vi "GetImage.vi"(0 "XRef":T4, 1 "State In":T3) -> (14 "Image":T2, 15 "Fatal Error Out":T1)   [LabVIEW 2015, in "Index JSON Array.xnode"]
uses:
  Index JSON Array.xnode
  <vilib>/XNodeSupport/XNodeXNodeRef.ctl
  State.ctl
  <vilib>/XNodeSupport/XNodeImage.ctl
  <vilib>/XNodeSupport/XNodeErrorCluster.ctl
  Build Array XNode/dimensions.vi
  Build Array XNode/Build JSON Array.xnode
  <vilib>/XNodeSupport/NI_XNodeSupport.lvlib
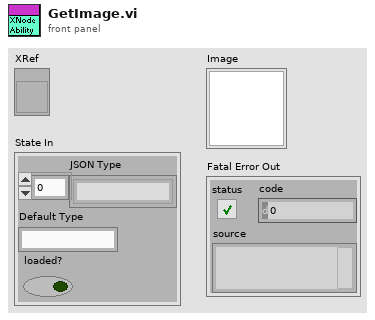
[diagram p1: front panel]
types:
  T1 = typedef "NI_XNodeSupport.lvlib/XNodeErrorCluster.ctl" = errorcluster
  T2 = typedef "NI_XNodeSupport.lvlib/XNodeImage.ctl" = picture
  T3 = typedef "Index JSON Array.xnode/State.ctl" = cluster{"JSON Type":string[], "Default Type":string, "loaded?":bool}
  T4 = typedef "NI_XNodeSupport.lvlib/XNodeXNodeRef.ctl" = refnum<vi>
  T5 = typedef "imagedata.ctl" = cluster{"image type":i32, "image depth":i32, "image":u8[], "mask":u8[], "colors":u32[], "Rectangle":cluster{"left":i16, "top":i16, "right":i16, "bottom":i16}}
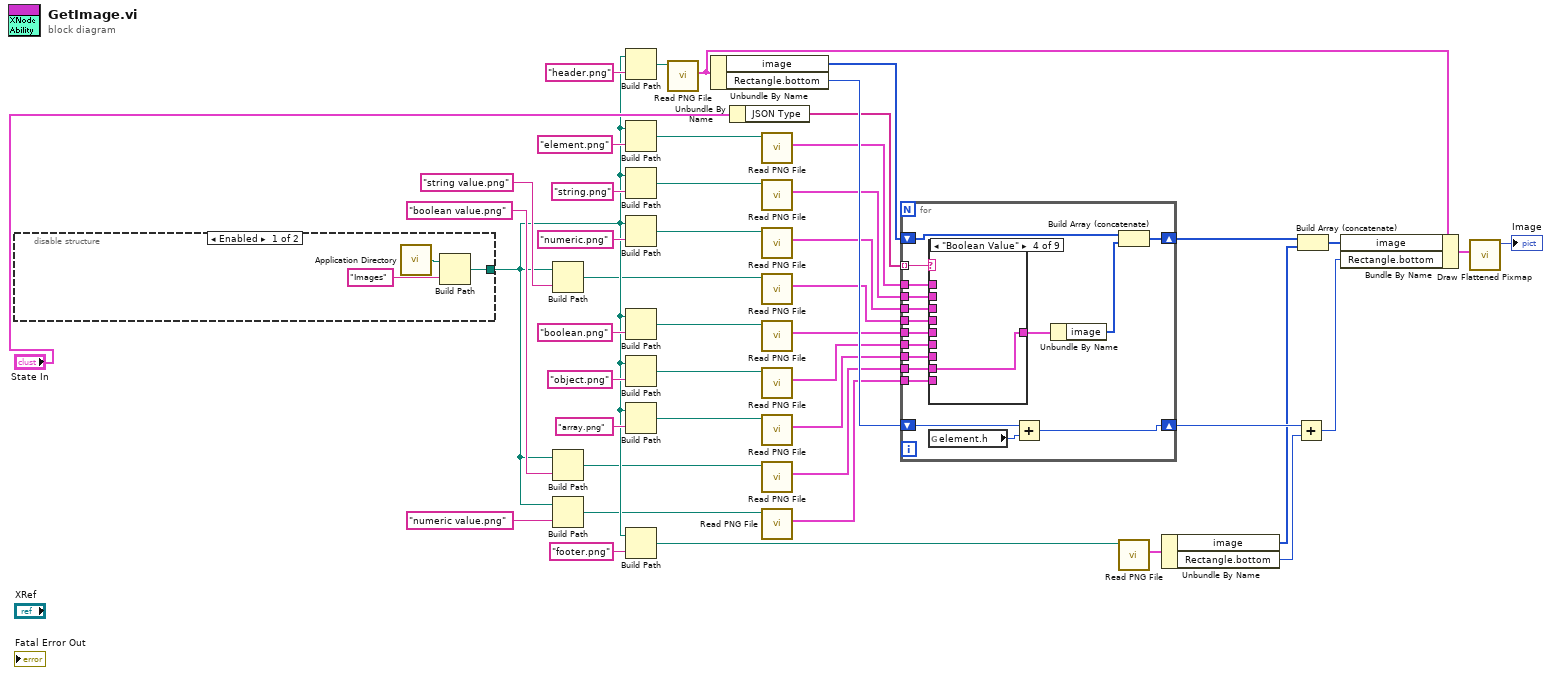
[diagram p0: block diagram]
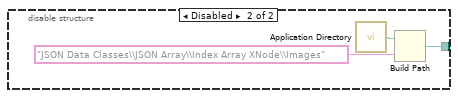
[diagram p10: hidden frame]
diagram:
  n1 = disable-structure shown="Enabled" {
    disable-tunnel: [w48 w51] -> w7
    frame Enabled {
      n2 = call <vilib>:"Application Directory.vi"() -> ("Application Directory"=w47:path)
      n3 = Build Path(base path=w47, name or relative path="Images") -> (appended path=w48:path)
    }
    frame Disabled {
      n4 = call <vilib>:"Application Directory.vi"() -> ("Application Directory"=w50:path)
      n5 = Build Path(base path=w50, name or relative path="JSON Data Classes\\JSON Array\\Index Array XNode\\Images") -> (appended path=w51:path)
    }
  }
  n6 = Build Path(base path=w7, name or relative path="string value.png") -> (appended path=w6:path)
  n7 = Build Path(base path=w7, name or relative path="boolean value.png") -> (appended path=w4:path)
  n8 = Build Path(base path=w7, name or relative path="numeric value.png") -> (appended path=w5:path)
  n9 = Build Path(base path=w7, name or relative path="header.png") -> (appended path=w42:path)
  n10 = Build Path(base path=w7, name or relative path="element.png") -> (appended path=w41:path)
  n11 = Build Path(base path=w7, name or relative path="string.png") -> (appended path=w25:path)
  n12 = Build Path(base path=w7, name or relative path="numeric.png") -> (appended path=w18:path)
  n13 = Build Path(base path=w7, name or relative path="boolean.png") -> (appended path=w16:path)
  n14 = Build Path(base path=w7, name or relative path="object.png") -> (appended path=w14:path)
  n15 = Build Path(base path=w7, name or relative path="array.png") -> (appended path=w15:path)
  n16 = Build Path(base path=w7, name or relative path="footer.png") -> (appended path=w40:path)
  n17 = call <vilib>:"Read PNG File.vi"("path to PNG file"=w42) -> ("image data"=w46:T5)  [unwired: 8 in, 2 out]
  n18 = Unbundle By Name(w46) -> ("image"=w38:u8[], "Rectangle.bottom"=w36:i16)
  n19 = Unbundle By Name("State In") -> ("JSON Type"=w27:string[])
  n20 = call <vilib>:"Read PNG File.vi"("path to PNG file"=w41) -> ("image data"=w23:T5)  [unwired: 8 in, 2 out]
  n21 = call <vilib>:"Read PNG File.vi"("path to PNG file"=w25) -> ("image data"=w24:T5)  [unwired: 8 in, 2 out]
  n22 = call <vilib>:"Read PNG File.vi"("path to PNG file"=w18) -> ("image data"=w17:T5)  [unwired: 8 in, 2 out]
  n23 = call <vilib>:"Read PNG File.vi"("path to PNG file"=w6) -> ("image data"=w3:T5)  [unwired: 8 in, 2 out]
  n24 = call <vilib>:"Read PNG File.vi"("path to PNG file"=w16) -> ("image data"=w13:T5)  [unwired: 8 in, 2 out]
  n25 = call <vilib>:"Read PNG File.vi"("path to PNG file"=w14) -> ("image data"=w11:T5)  [unwired: 8 in, 2 out]
  n26 = call <vilib>:"Read PNG File.vi"("path to PNG file"=w15) -> ("image data"=w12:T5)  [unwired: 8 in, 2 out]
  n27 = call <vilib>:"Read PNG File.vi"("path to PNG file"=w4) -> ("image data"=w1:T5)  [unwired: 8 in, 2 out]
  n28 = call <vilib>:"Read PNG File.vi"("path to PNG file"=w5) -> ("image data"=w2:T5)  [unwired: 8 in, 2 out]
  n29 = for {
    shift-right: [w65] -> w35
    shift-left: w38 -> [w69]
    shift-right: [w66] -> w33
    shift-left: w36 -> [w68]
    tunnel: w27 -> [w64] mode=indexing
    tunnel: w24 -> [w63]
    tunnel: w23 -> [w60]
    tunnel: w17 -> [w59]
    tunnel: w13 -> [w58]
    tunnel: w12 -> [w57]
    tunnel: w11 -> [w56]
    tunnel: w3 -> [w55]
    tunnel: w2 -> [w54]
    tunnel: w1 -> [w53]
    n30 = case shown="\"Boolean Value\"" w64 {
      tunnel: w63 -> [_ _ _ _ w74 _ _ _ _]
      tunnel: [w70 w71 w72 w73 w74 w75 w76 w77 w78] -> w62
      tunnel: w60 -> [w70 _ _ _ _ _ _ _ _]
      tunnel: w59 -> [_ _ _ _ _ w75 _ _ _]
      tunnel: w58 -> [_ _ _ _ _ _ w76 _ _]
      tunnel: w57 -> [_ _ _ _ _ _ _ w77 _]
      tunnel: w56 -> [_ _ _ _ _ _ _ _ w78]
      tunnel: w55 -> [_ w71 _ _ _ _ _ _ _]
      tunnel: w54 -> [_ _ w72 _ _ _ _ _ _]
      tunnel: w53 -> [_ _ _ w73 _ _ _ _ _]
      frame "JSON", Default {
      }
      frame "String Value" {
      }
      frame "Numeric Value" {
      }
      frame "Boolean Value" {
      }
      frame "JSON String" {
      }
      frame "JSON Numeric" {
      }
      frame "JSON Boolean" {
      }
      frame "JSON Array" {
      }
      frame "JSON Object" {
      }
    }
    n31 = global read "dimensions.vi" "element.h"() -> (w67:i16)
    n32 = Add(x=w68, y=w67) -> (x+y=w66:i16)
    n33 = Unbundle By Name(w62) -> ("image"=w61:u8[])
    n34 = Build Array (concatenate)(w69, w61) -> (w65:u8[])
  }
  n35 = call <vilib>:"Read PNG File.vi"("path to PNG file"=w40) -> ("image data"=w45:T5)  [unwired: 8 in, 2 out]
  n36 = Unbundle By Name(w45) -> ("image"=w32:u8[], "Rectangle.bottom"=w31:i16)
  n37 = Add(x=w33, y=w31) -> (x+y=w30:i16)
  n38 = Build Array (concatenate)(w35, w32) -> (w34:u8[])
  n39 = Bundle By Name(cluster=w46, "image"=w34, "Rectangle.bottom"=w30) -> (w37:T5)
  n40 = call <vilib>:"Draw Flattened Pixmap.vi"("image data"=w37) -> ("new picture"=→"Image":picture)  [unwired: 8 in]
